vi "Send_billede.vi"() -> ()   [LabVIEW 2018]
uses:
  <vilib>/myRIO/Instrument Drivers/Onboard IO/UART/typedef/VISA Configuration.ctl
  <vilib>/Instr/_visa.llb/VISA Configure Serial Port (Instr).vi
  <vilib>/myRIO/Express VI/Onboard IO/UART/UART Express VI.xnode
  <vilib>/myRIO/Instrument Drivers/Onboard IO/UART/UART.lvlib
panel:
  out "subarray":u8[][](array[numeric])
  out "array":u8[][](array[numeric])
  out "Intensity Graph 7":u8[][](graph)
  in  "Rotation \nOrientation 2":bool
  in  "stop":bool
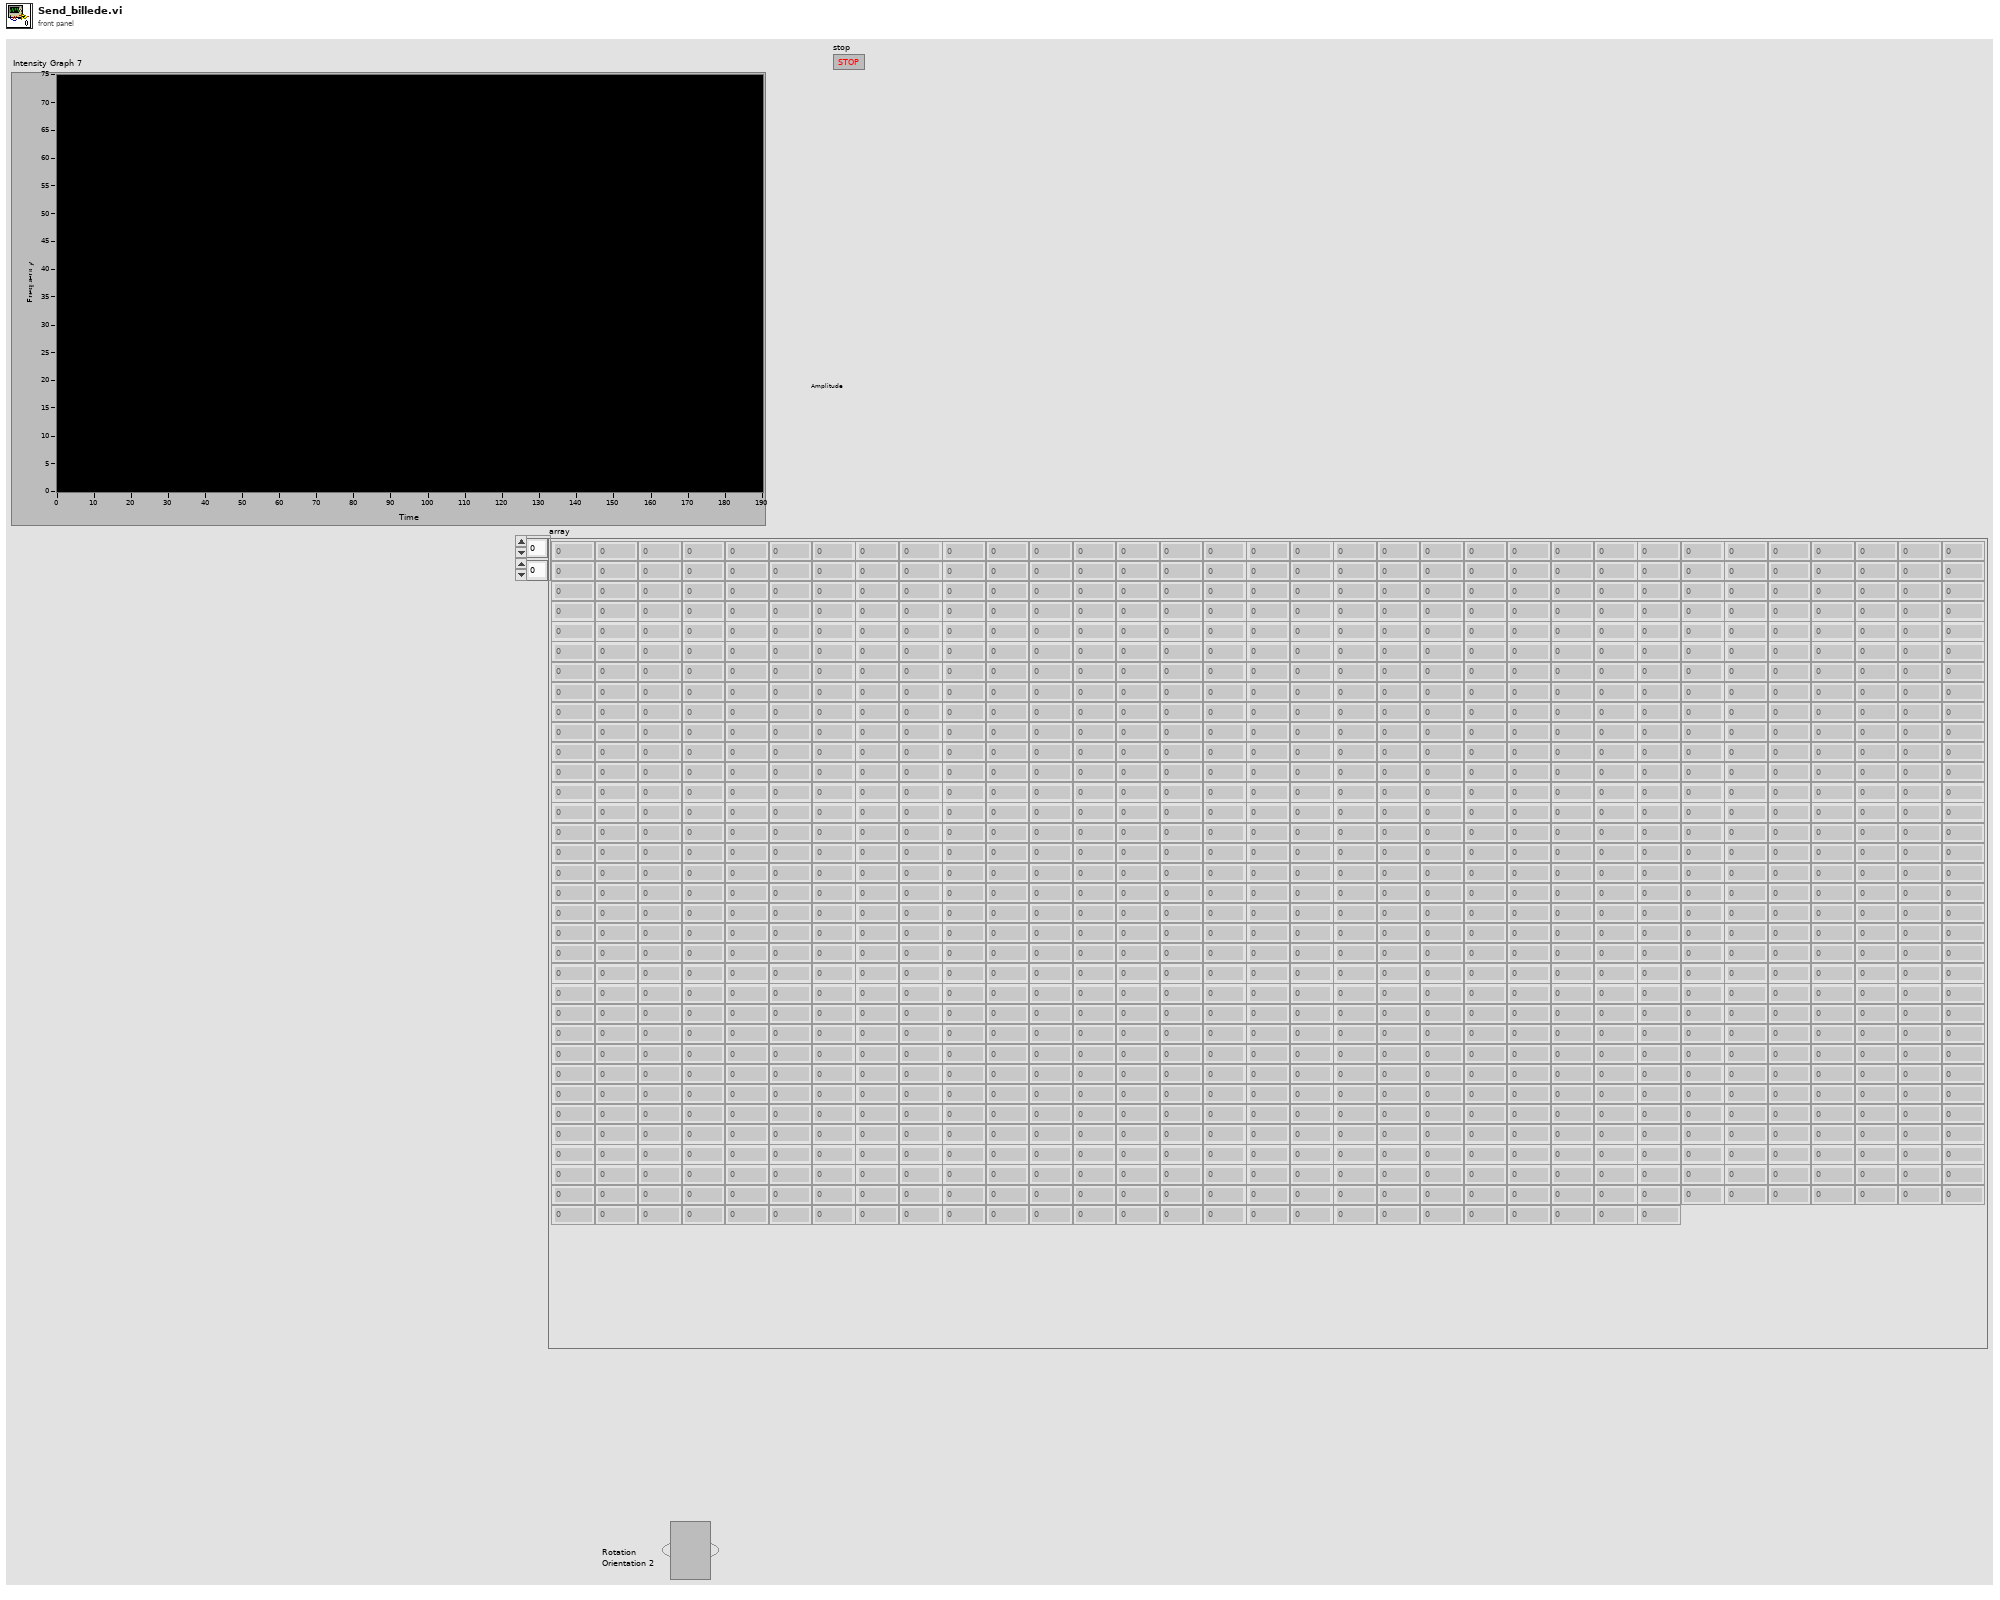
[diagram p1: front panel]
types:
  T1 = typedef "UART.lvlib/VISA Configuration.ctl" = cluster{"baud rate (9600)":u32, "data bits (8)":u16, "parity (0:none)":enum16{"None", "Odd", "Even", "Mark", "Space"}, "stop bits (10: 1 bit)":u16, "flow control (0:none)":u16, "termination char\n(0xA = '\\n' = LF) ":u8, "Enable Termination\nChar (T)":bool, "timeout (10sec)":u32}
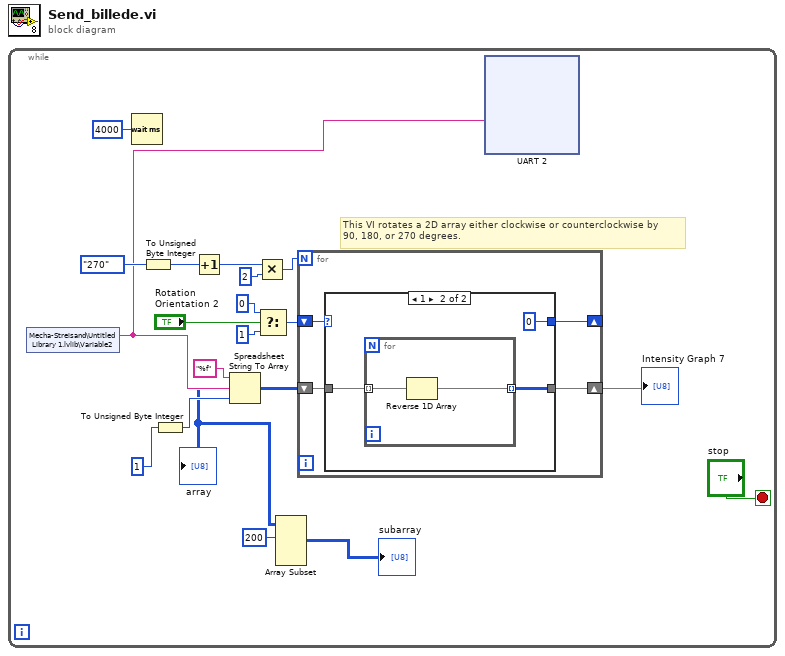
[diagram p0: block diagram]
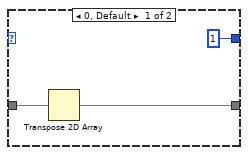
[diagram p2: hidden frame]
diagram:
  n1 = while {
    stop <- "stop" stop-if-true
    # "This VI rotates a 2D array either clockwise or counterclockwise by\n90, 180, or 270 degrees."
    n2 = shared-variable "Mecha-Streisand\\Untitled Library 1.lvlib\\Variable2"() -> (w4:string)  [unwired: 1 in, 1 out]
    n3 = Wait (ms)(milliseconds to wait=u32 4000) -> ()  [unwired: 1 out]
    n4 = To Unsigned Byte Integer(number=enum8{"90", "180", "270"}."270" ("Rotation")) -> (unsigned 8bit integer=w7:u8)
    n5 = To Unsigned Byte Integer(number=u8 1) -> (unsigned 8bit integer=w17:u8)
    n6 = Increment(x=w7) -> (x+1=w9:u8)
    n7 = Spreadsheet String To Array(format string="%f", spreadsheet string=w4, array type (2D Dbl)=w17) -> (array=w3:u8[][])  [unwired: 1 in]
    "array" <- w3
    n8 = Multiply(x=w9, y=u8 2) -> (x*y=w10:u8)
    n9 = Select(t=u8 0, s="Rotation \nOrientation 2", f=u8 1) -> (s? t:f=w11:u8)
    n10 = Array Subset(array=w3, index (row)=200 ("index")) -> (→"subarray":u8[][])  [unwired: 3 in]
    n11 = for {
      N: w10 -> [_]
      shift-right: [w38] -> w5
      shift-left: w3 -> [w39]
      shift-right: [w36] -> _
      shift-left: w11 -> [w37]
      n12 = case shown="1" w37 {
        tunnel: w39 -> [w41 w45]
        tunnel: [w42 w44] -> w38
        tunnel: [u8 1 u8 0] -> w36
        frame 0, Default {
          n13 = Transpose 2D Array(2D array=w41) -> (transposed array=w42:u8[][])
        }
        frame 1 {
          n14 = for {
            tunnel: w45 -> [w47] mode=indexing
            tunnel: [w46] -> w44 mode=indexing
            n15 = Reverse 1D Array(array=w47) -> (reversed array=w46:u8[])
          }
        }
      }
    }
    "Intensity Graph 7" <- w5
    n16 = xnode "UART 2"("Characters to Write"=w4) -> ()  [unwired: 1 in, 2 out]
  }
